vi "Normalize 2D Array.vi"(7 "Factor":i32, 9 "Maximum":dbl, 10 "Minimum":dbl, 11 "Array in":dbl[][](array[numeric])) -> (3 "Array out":dbl[][](array[numeric]))   [LabVIEW 2017, in "Measurement.PhotocurrentMapping.UI.lvclass"]
uses:
  Measurement.PhotocurrentMapping.UI.lvclass
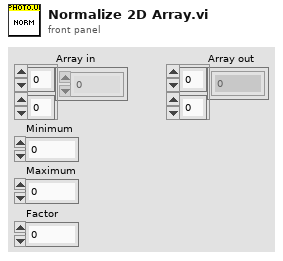
[diagram p1: front panel]
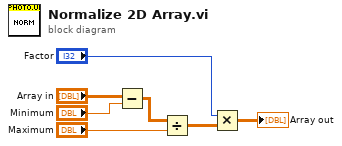
[diagram p0: block diagram]
diagram:
  n1 = Subtract(x="Array in", y="Minimum") -> (x-y=w3:dbl[][])
  n2 = Divide(x=w3, y="Maximum") -> (x/y=w5:dbl[][])
  n3 = Multiply(x="Factor", y=w5) -> (x*y=→"Array out":dbl[][])
